vi "Create.vi"(8 "error in":errorcluster, 11 "plugin references":T1) -> (0 "error out":errorcluster, 3 "fake measurement plugin":refnum<class "Fake Measurement Plugin.lvclass">)   [LabVIEW 2020, in "MeasurementServerTests.lvlib" / "Measurement Plugin Service Tests.lvlib" / "Fake Measurement Plugin.lvclass"]
uses:
  Fake Measurement Plugin.lvclass
  Plugin VI and Control References.ctl
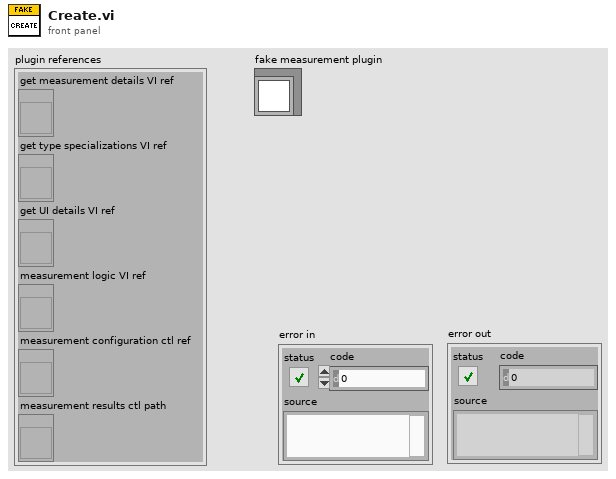
[diagram p1: front panel]
types:
  T1 = typedef "MeasurementServerTests.lvlib/Measurement Plugin Service Tests.lvlib/Fake Measurement Plugin.lvclass/Plugin VI and Control References.ctl" = cluster{"get measurement details VI ref":refnum<vi>, "get type specializations VI ref":refnum<vi>, "get UI details VI ref":refnum<vi>, "measurement logic VI ref":refnum<vi>, "measurement configuration ctl ref":refnum<vi>, "measurement results ctl path":refnum<vi>}
  T2 = cluster{"[0]":path, "[1]":path, "[2]":path, "[3]":path, "[4]":path, "[5]":path}
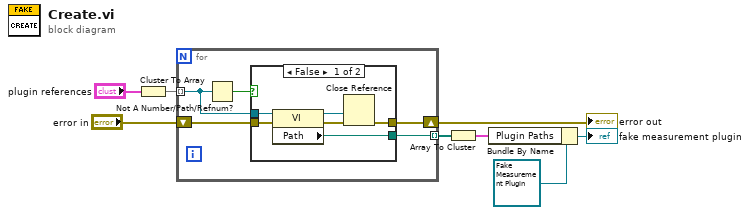
[diagram p0: block diagram]
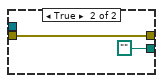
[diagram p2: hidden frame]
diagram:
  n1 = Cluster To Array(cluster="plugin references") -> (array=w5:refnum<vi>[])
  n2 = for {
    tunnel: w5 -> [w11] mode=indexing
    tunnel: [w12] -> w4 mode=indexing
    shift-right: [w10] -> w1
    shift-left: "error in" -> [w9]
    n3 = Not A Number/Path/Refnum?(number/path/refnum=w11) -> (NaN/Path/Refnum?=w13:bool)
    n4 = case shown="False" w13 {
      tunnel: [w18 path ""] -> w12
      tunnel: w11 -> [w19 _]
      tunnel: [w15 w20] -> w10
      tunnel: w9 -> [w14 w20]
      frame False {
        n5 = property class="VI"(reference=w19, error in=w14) -> (reference out=w17:refnum<vi>, error out=w16:errorcluster, "Path"=w18:path)
        n6 = Close Reference(reference=w17, error in (no error)=w16) -> (error out=w15:errorcluster)
      }
      frame True {
      }
    }
  }
  "error out" <- w1
  n7 = Array To Cluster(array=w4) -> (cluster=w3:T2)
  n8 = Bundle By Name(cluster=refnum<class "Fake Measurement Plugin.lvclass"> refnum ("MeasurementServerTests.lvlib:Measurement Plugin Service Tests.lvlib:Fake Measurement Plugin.lvclass"), "Plugin Paths"=w3) -> (→"fake measurement plugin":refnum<class "Fake Measurement Plugin.lvclass">)
